vi "Create Publisher.vi"(8 "error in (no error)":errorcluster, 9 "Default Value":dbl, 10 "Name":string, 11 "CIFTag in":refnum<class "CIFTagDouble.lvclass">) -> (0 "error out":errorcluster, 3 "CIFTag out":refnum<class "CIFTagDouble.lvclass">)   [LabVIEW 2021, in "CIFTagDouble.lvclass"]
uses:
  CIFTagDouble.lvclass
  D:/dev/CIF-LVCore/src/CIFUtilities/CIFChannels/CIFChannels.lvclass
  D:/dev/CIF-LVCore/src/Channels/CIFTag/CIFTag/CIFTag.lvclass
  CIFUtilities/CIFChannels/Typedef/Direction.ctl
  CIFUtilities/CIFChannels/Typedef/Disconnect Behavior.ctl
  CIFUtilities/CIFChannels/Typedef/Channel State.ctl
  CIFUtilities/CIFChannels/CIFChannels.lvclass/CIFChannels.ctl
  CIFTagDouble.lvclass/CIFTagDouble.ctl
  CIFTag/CIFTag.lvclass/CIFTag.ctl
  5c81bccc-e622-4fe9-9720-12299560a745.vi
  522c0ff3-de7b-4614-b37e-c276d07c7241.vi
  CIFUtilities/CIFChannels/Accessors/Write Channel State.vi
  CIFTag/Accessors/Write CIF Channel.vi
  CIFUtilities/CIFChannels/Accessors/Write Channel Class.vi
  CIFUtilities/CIFChannels/Accessors/Write Direction.vi
  CIFUtilities/CIFChannels/Accessors/Write Disconnect Behavior.vi
  CIFUtilities/CIFChannels/Accessors/Write Name.vi
  <vilib>/CIFChannels/SubVIs/Add Error.vi
  5c81bccc-e622-4fe9-9720-12299560a745.vi/c28b0ead-42ad-4072-80a2-aca7f2bd7ce3.vi
  <vilib>/CIFChannels/SubVIs/CIFServices Fill In Error Info Ex.vi
  <vilib>/CIFChannels/SubVIs/Get dll Path.vi
  522c0ff3-de7b-4614-b37e-c276d07c7241.vi/4bc1c15b-36ab-481f-b8dd-c64075ce723a.vi
  522c0ff3-de7b-4614-b37e-c276d07c7241.vi/d83cb72b-7713-41fc-a3d1-682de79cf574.vi
  <vilib>/CIFChannels/SubVIs/Append Error Location.vi
  CIFUtilities/CIFChannels/CIFChannels.lvclass
  D:/dev/CIF-LVCore/src/Channels/CIFTag/Double/CIFTagDouble.lvclass
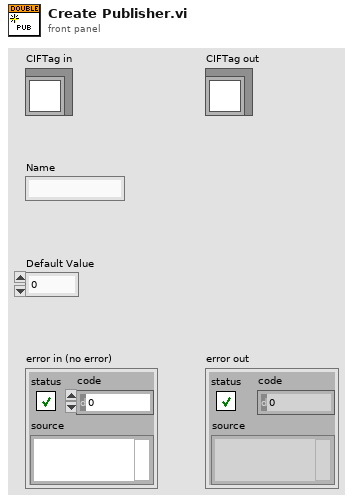
[diagram p1: front panel]
types:
  T1 = typedef "CIFChannels.lvclass/Channel State.ctl" = enum16{"Creating", "Disconnected", "Connecting", "Connected", "Destroying"}
  T2 = typedef "CIFChannels.lvclass/Disconnect Behavior.ctl" = enum16{"Default value", "Last value", "Error with default"}
  T3 = typedef "CIFChannels.lvclass/Direction.ctl" = enum16{"Publisher", "Subscriber"}
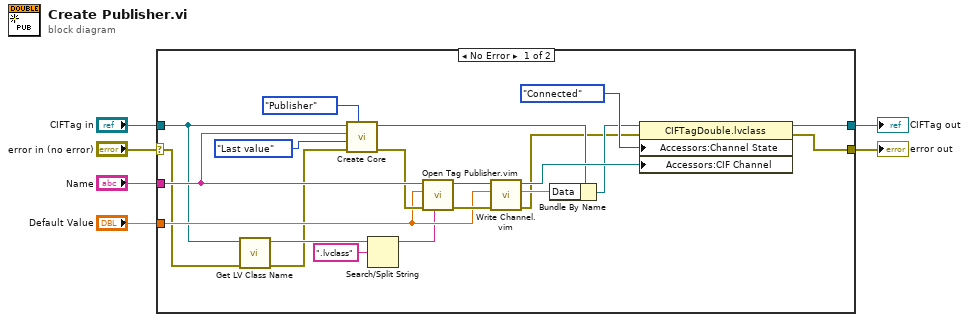
[diagram p0: block diagram]
diagram:
  n1 = case shown="No Error" "error in (no error)" {
    selector: "error in (no error)" -> [w8 w29]
    tunnel: [w24 w29] -> w5
    tunnel: [w13 w28] -> w3
    tunnel: "CIFTag in" -> [w12 w28]
    tunnel: "Name" -> [w23 _]
    tunnel: "Default Value" -> [w18 _]
    frame No Error {
      n2 = call <vilib>:"Get LV Class Name.vi"("error in (no error)"=w8, "object"=w12) -> ("error out"=w7:errorcluster, "class name"=w11:string)  [unwired: 8 in]
      n3 = call "Create Core.vi"("Direction"=Direction."Publisher", "error in (no error)"=w7, "Disconnect Behavior"=Disconnect_Behavior."Last value", "Name"=w23, "CIFChannels in"=w12) -> ("error out"=w22:errorcluster, "CIFChannels out"=w17:refnum<class "CIFTagDouble.lvclass">)  [unwired: 5 in]
      n4 = Search/Split String(string=w11, search string/char (-)=".lvclass") -> (substring before match=w9:string)  [unwired: 1 in, 2 out]
      n5 = call "Open Tag Publisher.vim"("Channel Type Description"=w9, "error in"=w22, "Input Type"=w18, "Channel Name"=w23) -> ("error out"=w20:errorcluster, "CIF Channel"=w21:refnum<k21>)  [unwired: 6 in]
      n6 = call "Write Channel.vim"("error in"=w20, "Data in"=w18, "CIF Channel in"=w21) -> ("error out"=w14:errorcluster, "Data out"=w15:dbl, "CIF Channel out"=w19:refnum<k21>)  [unwired: 5 in, 1 out]
      n7 = Bundle By Name(cluster=w17, "Data"=w15) -> (w16:refnum<class "CIFTagDouble.lvclass">)
      n8 = property class="CIFTagDouble.lvclass"(reference=w16, error in=w14, "Accessors:Channel State"=Channel_State."Connected" ("Channel State"), "Accessors:CIF Channel"=w19) -> (reference out=w13:refnum<class "CIFTagDouble.lvclass">, error out=w24:errorcluster)
    }
    frame Error {
    }
  }
  "error out" <- w5
  "CIFTag out" <- w3
